vi "LVObject to JSON.vi"(5 "enable LabVIEW extensions? (T)":bool=TRUE, 6 "Pretty Print?":bool, 7 "LVClass Serializer":refnum<class "Generic Object Serializer.lvclass">, 8 "error in (no error)":errorcluster, 10 "Object":refnum<class>) -> (0 "error out":errorcluster, 2 "<JSON>Object":string)   [LabVIEW 2017, in "Generic Object Serializer.lvclass"]
uses:
  Generic Object Serializer/Generic Object Serializer.lvclass
  C:/Program Files (x86)/National Instruments/LabVIEW 2017/vi.lib/JDP Science/JSONtext/LVClass Serializer/JSONtext LVClass Serializer.lvclass
  <vilib>/PNR/LabVIEW Composition/Composition/Composition.lvlib
  <vilib>/JDP Science/JSONtext/JSONtext.lvlib
  <vilib>/JDP Science/JDP Science Common Utilities/JDP Utility.lvlib
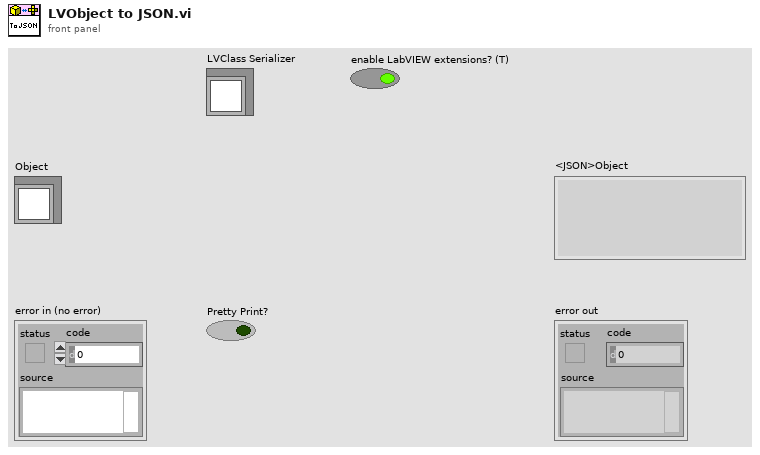
[diagram p1: front panel]
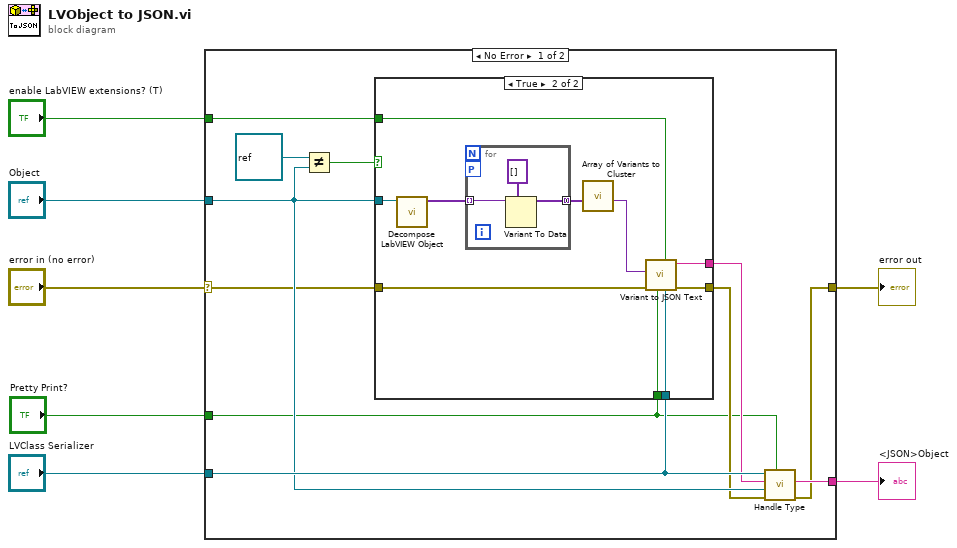
[diagram p0: block diagram]
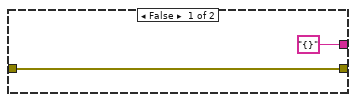
[diagram p2: hidden frame]
diagram:
  n1 = case shown="No Error" "error in (no error)" {
    selector: "error in (no error)" -> [w11 w34]
    tunnel: "Object" -> [w15 _]
    tunnel: [w13 _] -> w6
    tunnel: "LVClass Serializer" -> [w16 _]
    tunnel: [w9 w34] -> w3
    tunnel: "enable LabVIEW extensions? (T)" -> [w12 _]
    tunnel: "Pretty Print?" -> [w8 _]
    frame No Error {
      n2 = Not Equal?(x=refnum<class> refnum, y=w15) -> (x != y?=w17:bool)
      n3 = case shown="True" w17 {
        tunnel: ["{}" ("<JSON>") w29] -> w14
        tunnel: w15 -> [_ w30]
        tunnel: w16 -> [_ w28]
        tunnel: w12 -> [_ w27]
        tunnel: [w19 w23] -> w10
        tunnel: w11 -> [w19 w22]
        tunnel: w8 -> [_ w21]
        frame False {
        }
        frame True {
          n4 = call <vilib>:"Decompose LabVIEW Object.vi"("LabVIEW Object"=w30) -> ("Private Data Clusters"=w25:variant[])  [unwired: 7 in, 3 out]
          n5 = for {
            tunnel: w25 -> [w33] mode=indexing
            tunnel: [w31] -> w26 mode=concatenating
            workers-P: _ -> [_]
            n6 = Variant To Data(type=variant[] [], Variant=w33) -> (data=w31:variant[])  [unwired: 1 in, 1 out]
          }
          n7 = call <vilib>:"Array of Variants to Cluster.vi"("Array of Variants"=w26) -> ("Cluster of Variants"=w24:variant)  [unwired: 10 in]
          n8 = call <vilib>:"Variant to JSON Text.vi"("LVClass Serializer"=w28, "enable LabVIEW extensions? (T)"=w27, "Pretty Print?"=w21, "error in (no error)"=w22, "Variant"=w24) -> ("error out"=w23:errorcluster, "<JSON>"=w29:string)  [unwired: 4 in, 1 out]
        }
      }
      n9 = call "Handle Type.vi"("Pretty Print?"=w8, "error in (no error)"=w10, "Type"=w15, "JSON"=w14, "Flatten To JSON Object in"=w16) -> ("error out"=w9:errorcluster, "JSON out"=w13:string)  [unwired: 4 in, 1 out]
    }
    frame Error {
    }
  }
  "error out" <- w3
  "<JSON>Object" <- w6
